vi "SequenceSelector_Load.vi"(0 "Ring 8":bool, 1 "Ring 7":bool, 2 "Ring 6":bool, 3 "Ring 5":bool, 4 "Loop Iteration":i32, 5 "Inflow Channel Selector":dbl, 7 "Ring 4":bool, 8 "Ring 3":bool, 9 "Ring 2":bool, 10 "Ring 1":bool) -> (6 "Array":u8[][](array[numeric])=[[0, 0, 0, 0, 0, 0, 0, 0, 2, 4, 3, 3, 3, 3], [0, 0, 0, 0, 0, 0, 0, 0, 0, 0, 0, 0, 0, 0], [0, 0, 0, 0, 0, 0, 0, 0, 0, 0, 0, 0, 0, 0], [0, 0, 0, 0, 0, 0, 0, 0, 0, 0, 0, 0, 0, 0], [0, 0, 0, 0, 0, 0, 0, 0, 0, 0, 0, 0, 0, 0], [11, 11, 11, 11, 11, 11, 11, 0, 0, 0, 0, 0, 0, 0], [0, 0, 0, 0, 0, 0, 0, 0, 0, 0, 0, 0, 0, 0], [16, 16, 16, 16, 16, 16, 16, 0, 0, 0, 0, 0, 0, 0], [0, 0, 0, 0, 0, 0, 0, 0, 0, 0, 0, 0, 0, 0], [0, 0, 0, 0, 0, 0, 0, 0, 0, 0, 0, 0, 0, 0], [0, 0, 0, 0, 0, 0, 0, 0, 0, 0, 0, 0, 0, 0], [2, 2, 2, 2, 2, 2, 2, 0, 0, 0, 0, 0, 0, 0], [4, 4, 4, 4, 4, 4, 4, 0, 0, 0, 0, 0, 0, 0], [255, 255, 255, 255, 255, 255, 0, 0, 0, 0, 0, 0, 0, 0], [3, 2, 6, 4, 5, 1, 0, 0, 0, 0, 0, 0, 0, 0], [31, 31, 31, 31, 31, 31, 0, 0, 0, 0, 0, 0, 0, 0], [255, 255, 255, 255, 255, 255, 0, 0, 0, 0, 0, 0, 0, 0]])   [LabVIEW 2016]
panel:
  in  "Byte 4":dbl[](array[numeric])
  in  "Byte 3":dbl[](array[numeric])
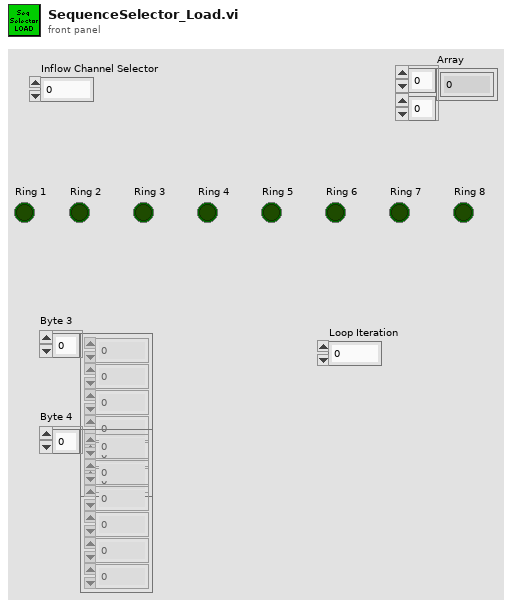
[diagram p1: front panel]
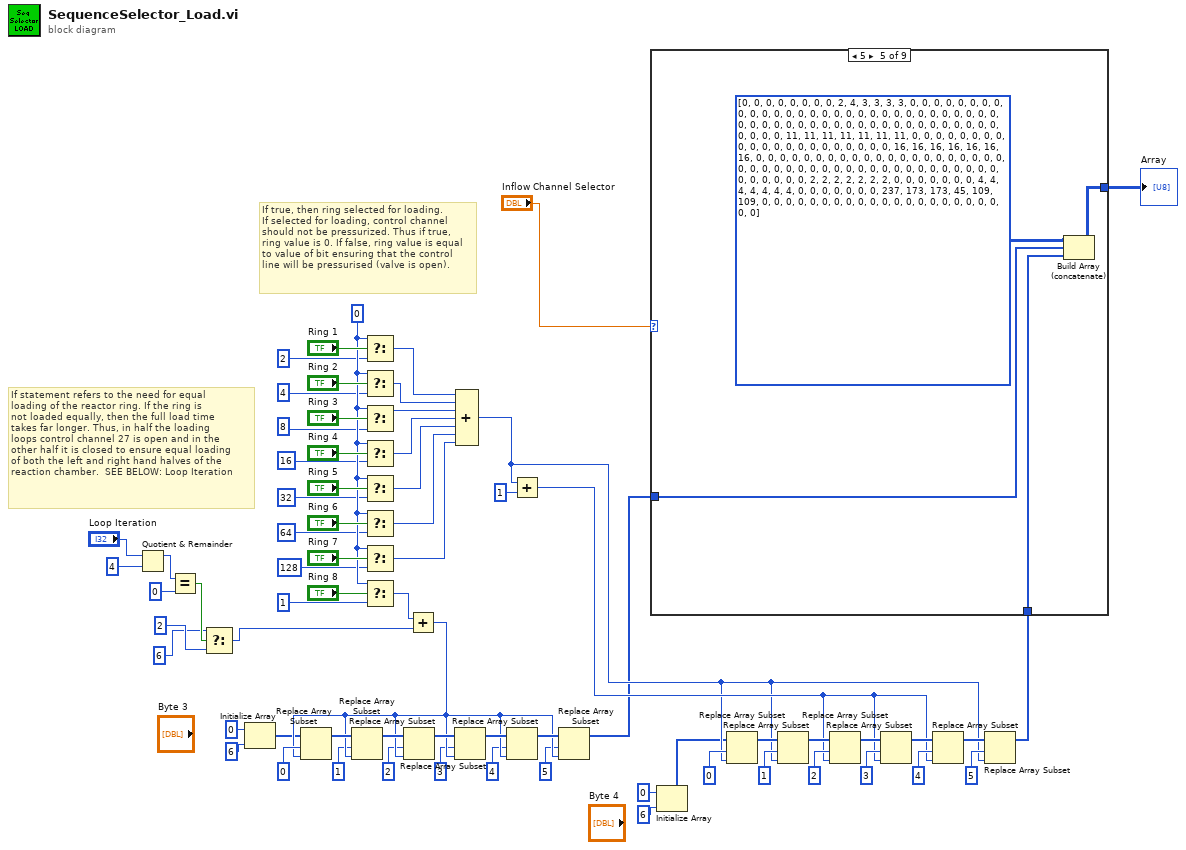
[diagram p0: block diagram]
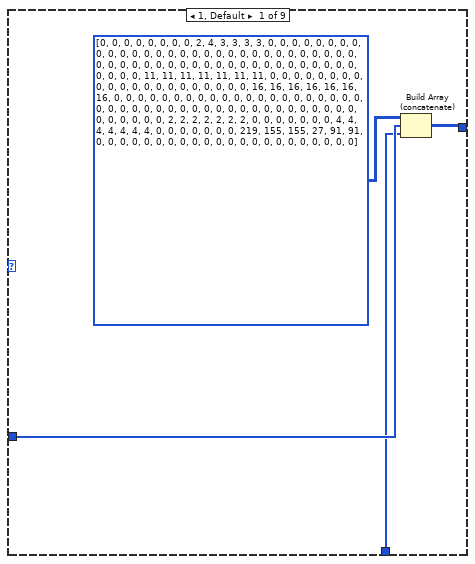
[diagram p2: hidden frame]
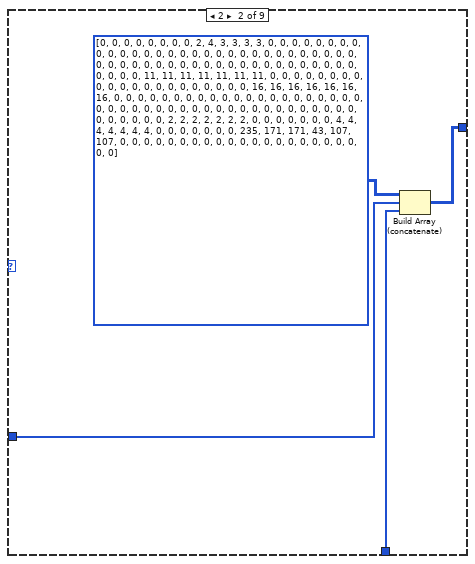
[diagram p3: hidden frame]
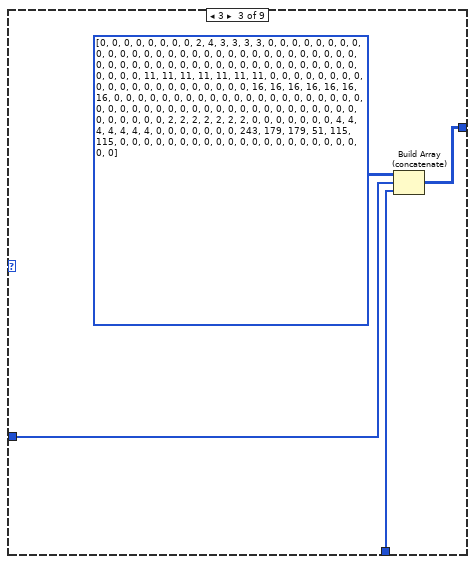
[diagram p4: hidden frame]
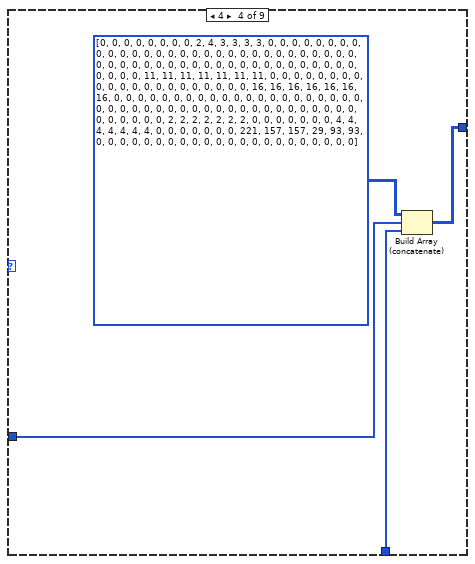
[diagram p5: hidden frame]
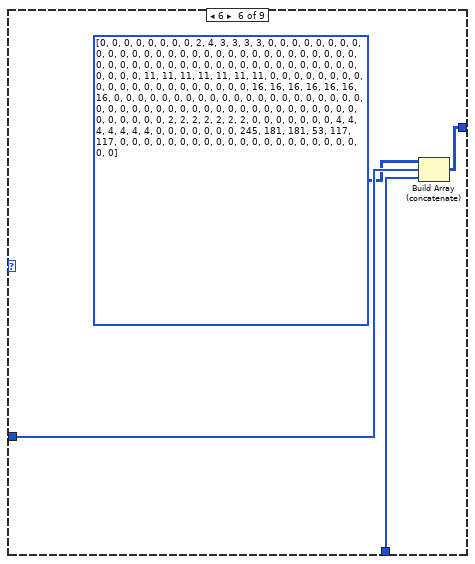
[diagram p6: hidden frame]
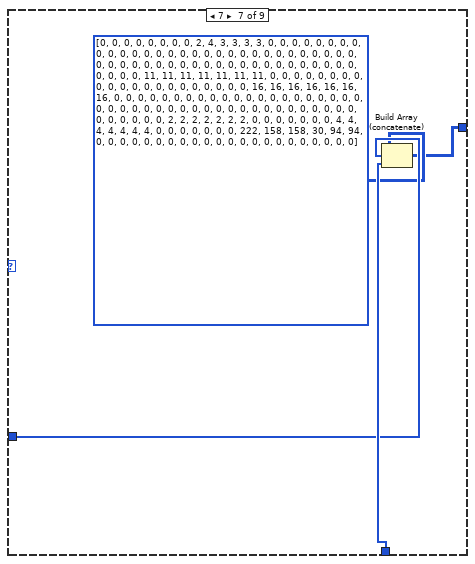
[diagram p7: hidden frame]
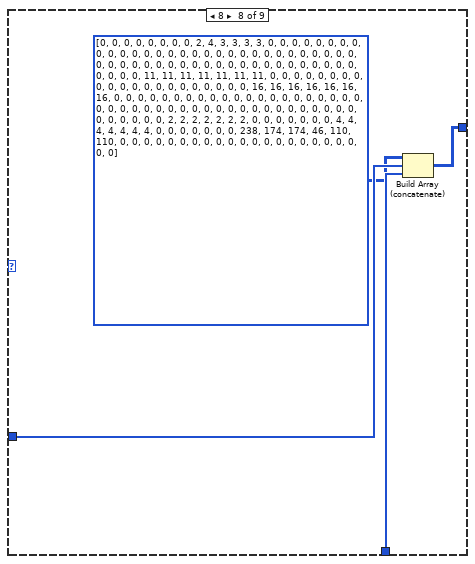
[diagram p8: hidden frame]
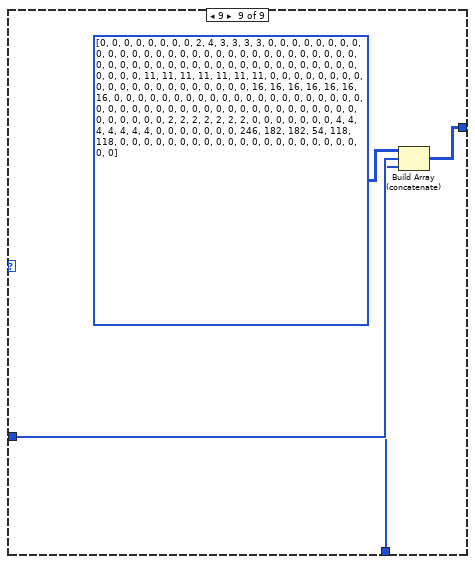
[diagram p9: hidden frame]
diagram:
  w60 = 0
  # "If statement refers to the need for equal \nloading of the reactor ring. If the ring is \nnot loaded equally, then the full load time \ntakes far longer. Thus, in half the loading\nloops control channel 27 is open and in the\nother half it is closed to ensure equal loading\nof both the left and right hand halves of the \nreaction chamber.  SEE BELOW: Loop Iteration"
  # "If true, then ring selected for loading. \nIf selected for loading, control channel\nshould not be pressurized. Thus if true, \nring value is 0. If false, ring value is equal\nto value of bit ensuring that the control \nline will be pressurised (valve is open)."
  n1 = Quotient & Remainder(x="Loop Iteration", y=4) -> (x-y*floor(x/y)=w4:i32)  [unwired: 1 out]
  n2 = Equal?(x=w4, y=0) -> (x = y?=w7:bool)
  n3 = Select(t=6, s=w7, f=2) -> (s? t:f=w8:i32)
  n4 = Initialize Array(0, 6) -> (w9:i32[])
  n5 = Select(t=w60, s="Ring 1", f=2) -> (s? t:f=w27:i32)
  n6 = Select(t=w60, s="Ring 2", f=4) -> (s? t:f=w26:i32)
  n7 = Select(t=w60, s="Ring 3", f=8) -> (s? t:f=w25:i32)
  n8 = Select(t=w60, s="Ring 4", f=16) -> (s? t:f=w24:i32)
  n9 = Select(t=w60, s="Ring 5", f=32) -> (s? t:f=w23:i32)
  n10 = Select(t=w60, s="Ring 6", f=64) -> (s? t:f=w22:i32)
  n11 = Select(t=w60, s="Ring 7", f=128) -> (s? t:f=w21:i32)
  n12 = Select(t=w60, s="Ring 8", f=1) -> (s? t:f=w51:i32)
  n13 = Add(x=w51, y=w8) -> (x+y=w44:i32)
  n14 = Replace Array Subset(array=w9, new element=w44, index=0) -> (w49:i32[])
  n15 = Replace Array Subset(array=w49, new element=w44, index=1) -> (w48:i32[])
  n16 = Replace Array Subset(array=w48, new element=w44, index=2) -> (w47:i32[])
  n17 = Replace Array Subset(array=w47, new element=w44, index=3) -> (w46:i32[])
  n18 = Compound Arithmetic op=ADD(w27, w26, w25, w24, w23, w22, w21) -> (w18:i32)
  n19 = Replace Array Subset(array=w46, new element=w44, index=4) -> (w45:i32[])
  n20 = Add(x=w18, y=1) -> (x+y=w19:i32)
  n21 = Replace Array Subset(array=w45, new element=w44, index=5) -> (w17:i32[])
  n22 = Initialize Array(0, 6) -> (w14:i32[])
  n23 = Replace Array Subset(array=w14, new element=w18, index=0) -> (w29:i32[])
  n24 = Replace Array Subset(array=w29, new element=w18, index=1) -> (w30:i32[])
  n25 = Replace Array Subset(array=w30, new element=w19, index=2) -> (w31:i32[])
  n26 = Replace Array Subset(array=w31, new element=w19, index=3) -> (w32:i32[])
  n27 = Replace Array Subset(array=w32, new element=w19, index=4) -> (w33:i32[])
  n28 = Replace Array Subset(array=w33, new element=w18, index=5) -> (w16:i32[])
  n29 = case shown="5" "Inflow Channel Selector" {
    tunnel: [w73 w74 w78 w82 w89 w93 w94 w98 w104] -> w15
    tunnel: w17 -> [w71 w76 w80 w84 w87 w91 w96 w100 w103]
    tunnel: w16 -> [w70 w77 w81 w85 w88 w92 w97 w101 w102]
    frame 1, Default {
      n30 = Build Array (concatenate)(u8[][] [[0, 0, 0, 0, 0, 0, 0, 0, 2, 4, 3, 3, 3, 3], [0, 0, 0, 0, 0, 0, 0, 0, 0, 0, 0, 0, 0, 0], [0, 0, 0, 0, 0, 0, 0, 0, 0, 0, 0, 0, 0, 0], [0, 0, 0, 0, 0, 0, 0, 0, 0, 0, 0, 0, 0, 0], [0, 0, 0, 0, 0, 0, 0, 0, 0, 0, 0, 0, 0, 0], [11, 11, 11, 11, 11, 11, 11, 0, 0, 0, 0, 0, 0, 0], [0, 0, 0, 0, 0, 0, 0, 0, 0, 0, 0, 0, 0, 0], [16, 16, 16, 16, 16, 16, 16, 0, 0, 0, 0, 0, 0, 0], [0, 0, 0, 0, 0, 0, 0, 0, 0, 0, 0, 0, 0, 0], [0, 0, 0, 0, 0, 0, 0, 0, 0, 0, 0, 0, 0, 0], [0, 0, 0, 0, 0, 0, 0, 0, 0, 0, 0, 0, 0, 0], [2, 2, 2, 2, 2, 2, 2, 0, 0, 0, 0, 0, 0, 0], [4, 4, 4, 4, 4, 4, 4, 0, 0, 0, 0, 0, 0, 0], [219, 155, 155, 27, 91, 91, 0, 0, 0, 0, 0, 0, 0, 0], [0, 0, 0, 0, 0, 0, 0, 0, 0, 0, 0, 0, 0, 0]], w71, w70) -> (w73:i32[][])
    }
    frame 2 {
      n31 = Build Array (concatenate)(u8[][] [[0, 0, 0, 0, 0, 0, 0, 0, 2, 4, 3, 3, 3, 3], [0, 0, 0, 0, 0, 0, 0, 0, 0, 0, 0, 0, 0, 0], [0, 0, 0, 0, 0, 0, 0, 0, 0, 0, 0, 0, 0, 0], [0, 0, 0, 0, 0, 0, 0, 0, 0, 0, 0, 0, 0, 0], [0, 0, 0, 0, 0, 0, 0, 0, 0, 0, 0, 0, 0, 0], [11, 11, 11, 11, 11, 11, 11, 0, 0, 0, 0, 0, 0, 0], [0, 0, 0, 0, 0, 0, 0, 0, 0, 0, 0, 0, 0, 0], [16, 16, 16, 16, 16, 16, 16, 0, 0, 0, 0, 0, 0, 0], [0, 0, 0, 0, 0, 0, 0, 0, 0, 0, 0, 0, 0, 0], [0, 0, 0, 0, 0, 0, 0, 0, 0, 0, 0, 0, 0, 0], [0, 0, 0, 0, 0, 0, 0, 0, 0, 0, 0, 0, 0, 0], [2, 2, 2, 2, 2, 2, 2, 0, 0, 0, 0, 0, 0, 0], [4, 4, 4, 4, 4, 4, 4, 0, 0, 0, 0, 0, 0, 0], [235, 171, 171, 43, 107, 107, 0, 0, 0, 0, 0, 0, 0, 0], [0, 0, 0, 0, 0, 0, 0, 0, 0, 0, 0, 0, 0, 0]], w76, w77) -> (w74:i32[][])
    }
    frame 3 {
      n32 = Build Array (concatenate)(u8[][] [[0, 0, 0, 0, 0, 0, 0, 0, 2, 4, 3, 3, 3, 3], [0, 0, 0, 0, 0, 0, 0, 0, 0, 0, 0, 0, 0, 0], [0, 0, 0, 0, 0, 0, 0, 0, 0, 0, 0, 0, 0, 0], [0, 0, 0, 0, 0, 0, 0, 0, 0, 0, 0, 0, 0, 0], [0, 0, 0, 0, 0, 0, 0, 0, 0, 0, 0, 0, 0, 0], [11, 11, 11, 11, 11, 11, 11, 0, 0, 0, 0, 0, 0, 0], [0, 0, 0, 0, 0, 0, 0, 0, 0, 0, 0, 0, 0, 0], [16, 16, 16, 16, 16, 16, 16, 0, 0, 0, 0, 0, 0, 0], [0, 0, 0, 0, 0, 0, 0, 0, 0, 0, 0, 0, 0, 0], [0, 0, 0, 0, 0, 0, 0, 0, 0, 0, 0, 0, 0, 0], [0, 0, 0, 0, 0, 0, 0, 0, 0, 0, 0, 0, 0, 0], [2, 2, 2, 2, 2, 2, 2, 0, 0, 0, 0, 0, 0, 0], [4, 4, 4, 4, 4, 4, 4, 0, 0, 0, 0, 0, 0, 0], [243, 179, 179, 51, 115, 115, 0, 0, 0, 0, 0, 0, 0, 0], [0, 0, 0, 0, 0, 0, 0, 0, 0, 0, 0, 0, 0, 0]], w80, w81) -> (w78:i32[][])
    }
    frame 4 {
      n33 = Build Array (concatenate)(u8[][] [[0, 0, 0, 0, 0, 0, 0, 0, 2, 4, 3, 3, 3, 3], [0, 0, 0, 0, 0, 0, 0, 0, 0, 0, 0, 0, 0, 0], [0, 0, 0, 0, 0, 0, 0, 0, 0, 0, 0, 0, 0, 0], [0, 0, 0, 0, 0, 0, 0, 0, 0, 0, 0, 0, 0, 0], [0, 0, 0, 0, 0, 0, 0, 0, 0, 0, 0, 0, 0, 0], [11, 11, 11, 11, 11, 11, 11, 0, 0, 0, 0, 0, 0, 0], [0, 0, 0, 0, 0, 0, 0, 0, 0, 0, 0, 0, 0, 0], [16, 16, 16, 16, 16, 16, 16, 0, 0, 0, 0, 0, 0, 0], [0, 0, 0, 0, 0, 0, 0, 0, 0, 0, 0, 0, 0, 0], [0, 0, 0, 0, 0, 0, 0, 0, 0, 0, 0, 0, 0, 0], [0, 0, 0, 0, 0, 0, 0, 0, 0, 0, 0, 0, 0, 0], [2, 2, 2, 2, 2, 2, 2, 0, 0, 0, 0, 0, 0, 0], [4, 4, 4, 4, 4, 4, 4, 0, 0, 0, 0, 0, 0, 0], [221, 157, 157, 29, 93, 93, 0, 0, 0, 0, 0, 0, 0, 0], [0, 0, 0, 0, 0, 0, 0, 0, 0, 0, 0, 0, 0, 0]], w84, w85) -> (w82:i32[][])
    }
    frame 5 {
      n34 = Build Array (concatenate)(u8[][] [[0, 0, 0, 0, 0, 0, 0, 0, 2, 4, 3, 3, 3, 3], [0, 0, 0, 0, 0, 0, 0, 0, 0, 0, 0, 0, 0, 0], [0, 0, 0, 0, 0, 0, 0, 0, 0, 0, 0, 0, 0, 0], [0, 0, 0, 0, 0, 0, 0, 0, 0, 0, 0, 0, 0, 0], [0, 0, 0, 0, 0, 0, 0, 0, 0, 0, 0, 0, 0, 0], [11, 11, 11, 11, 11, 11, 11, 0, 0, 0, 0, 0, 0, 0], [0, 0, 0, 0, 0, 0, 0, 0, 0, 0, 0, 0, 0, 0], [16, 16, 16, 16, 16, 16, 16, 0, 0, 0, 0, 0, 0, 0], [0, 0, 0, 0, 0, 0, 0, 0, 0, 0, 0, 0, 0, 0], [0, 0, 0, 0, 0, 0, 0, 0, 0, 0, 0, 0, 0, 0], [0, 0, 0, 0, 0, 0, 0, 0, 0, 0, 0, 0, 0, 0], [2, 2, 2, 2, 2, 2, 2, 0, 0, 0, 0, 0, 0, 0], [4, 4, 4, 4, 4, 4, 4, 0, 0, 0, 0, 0, 0, 0], [237, 173, 173, 45, 109, 109, 0, 0, 0, 0, 0, 0, 0, 0], [0, 0, 0, 0, 0, 0, 0, 0, 0, 0, 0, 0, 0, 0]], w87, w88) -> (w89:i32[][])
    }
    frame 6 {
      n35 = Build Array (concatenate)(u8[][] [[0, 0, 0, 0, 0, 0, 0, 0, 2, 4, 3, 3, 3, 3], [0, 0, 0, 0, 0, 0, 0, 0, 0, 0, 0, 0, 0, 0], [0, 0, 0, 0, 0, 0, 0, 0, 0, 0, 0, 0, 0, 0], [0, 0, 0, 0, 0, 0, 0, 0, 0, 0, 0, 0, 0, 0], [0, 0, 0, 0, 0, 0, 0, 0, 0, 0, 0, 0, 0, 0], [11, 11, 11, 11, 11, 11, 11, 0, 0, 0, 0, 0, 0, 0], [0, 0, 0, 0, 0, 0, 0, 0, 0, 0, 0, 0, 0, 0], [16, 16, 16, 16, 16, 16, 16, 0, 0, 0, 0, 0, 0, 0], [0, 0, 0, 0, 0, 0, 0, 0, 0, 0, 0, 0, 0, 0], [0, 0, 0, 0, 0, 0, 0, 0, 0, 0, 0, 0, 0, 0], [0, 0, 0, 0, 0, 0, 0, 0, 0, 0, 0, 0, 0, 0], [2, 2, 2, 2, 2, 2, 2, 0, 0, 0, 0, 0, 0, 0], [4, 4, 4, 4, 4, 4, 4, 0, 0, 0, 0, 0, 0, 0], [245, 181, 181, 53, 117, 117, 0, 0, 0, 0, 0, 0, 0, 0], [0, 0, 0, 0, 0, 0, 0, 0, 0, 0, 0, 0, 0, 0]], w91, w92) -> (w93:i32[][])
    }
    frame 7 {
      n36 = Build Array (concatenate)(u8[][] [[0, 0, 0, 0, 0, 0, 0, 0, 2, 4, 3, 3, 3, 3], [0, 0, 0, 0, 0, 0, 0, 0, 0, 0, 0, 0, 0, 0], [0, 0, 0, 0, 0, 0, 0, 0, 0, 0, 0, 0, 0, 0], [0, 0, 0, 0, 0, 0, 0, 0, 0, 0, 0, 0, 0, 0], [0, 0, 0, 0, 0, 0, 0, 0, 0, 0, 0, 0, 0, 0], [11, 11, 11, 11, 11, 11, 11, 0, 0, 0, 0, 0, 0, 0], [0, 0, 0, 0, 0, 0, 0, 0, 0, 0, 0, 0, 0, 0], [16, 16, 16, 16, 16, 16, 16, 0, 0, 0, 0, 0, 0, 0], [0, 0, 0, 0, 0, 0, 0, 0, 0, 0, 0, 0, 0, 0], [0, 0, 0, 0, 0, 0, 0, 0, 0, 0, 0, 0, 0, 0], [0, 0, 0, 0, 0, 0, 0, 0, 0, 0, 0, 0, 0, 0], [2, 2, 2, 2, 2, 2, 2, 0, 0, 0, 0, 0, 0, 0], [4, 4, 4, 4, 4, 4, 4, 0, 0, 0, 0, 0, 0, 0], [222, 158, 158, 30, 94, 94, 0, 0, 0, 0, 0, 0, 0, 0], [0, 0, 0, 0, 0, 0, 0, 0, 0, 0, 0, 0, 0, 0]], w96, w97) -> (w94:i32[][])
    }
    frame 8 {
      n37 = Build Array (concatenate)(u8[][] [[0, 0, 0, 0, 0, 0, 0, 0, 2, 4, 3, 3, 3, 3], [0, 0, 0, 0, 0, 0, 0, 0, 0, 0, 0, 0, 0, 0], [0, 0, 0, 0, 0, 0, 0, 0, 0, 0, 0, 0, 0, 0], [0, 0, 0, 0, 0, 0, 0, 0, 0, 0, 0, 0, 0, 0], [0, 0, 0, 0, 0, 0, 0, 0, 0, 0, 0, 0, 0, 0], [11, 11, 11, 11, 11, 11, 11, 0, 0, 0, 0, 0, 0, 0], [0, 0, 0, 0, 0, 0, 0, 0, 0, 0, 0, 0, 0, 0], [16, 16, 16, 16, 16, 16, 16, 0, 0, 0, 0, 0, 0, 0], [0, 0, 0, 0, 0, 0, 0, 0, 0, 0, 0, 0, 0, 0], [0, 0, 0, 0, 0, 0, 0, 0, 0, 0, 0, 0, 0, 0], [0, 0, 0, 0, 0, 0, 0, 0, 0, 0, 0, 0, 0, 0], [2, 2, 2, 2, 2, 2, 2, 0, 0, 0, 0, 0, 0, 0], [4, 4, 4, 4, 4, 4, 4, 0, 0, 0, 0, 0, 0, 0], [238, 174, 174, 46, 110, 110, 0, 0, 0, 0, 0, 0, 0, 0], [0, 0, 0, 0, 0, 0, 0, 0, 0, 0, 0, 0, 0, 0]], w100, w101) -> (w98:i32[][])
    }
    frame 9 {
      n38 = Build Array (concatenate)(u8[][] [[0, 0, 0, 0, 0, 0, 0, 0, 2, 4, 3, 3, 3, 3], [0, 0, 0, 0, 0, 0, 0, 0, 0, 0, 0, 0, 0, 0], [0, 0, 0, 0, 0, 0, 0, 0, 0, 0, 0, 0, 0, 0], [0, 0, 0, 0, 0, 0, 0, 0, 0, 0, 0, 0, 0, 0], [0, 0, 0, 0, 0, 0, 0, 0, 0, 0, 0, 0, 0, 0], [11, 11, 11, 11, 11, 11, 11, 0, 0, 0, 0, 0, 0, 0], [0, 0, 0, 0, 0, 0, 0, 0, 0, 0, 0, 0, 0, 0], [16, 16, 16, 16, 16, 16, 16, 0, 0, 0, 0, 0, 0, 0], [0, 0, 0, 0, 0, 0, 0, 0, 0, 0, 0, 0, 0, 0], [0, 0, 0, 0, 0, 0, 0, 0, 0, 0, 0, 0, 0, 0], [0, 0, 0, 0, 0, 0, 0, 0, 0, 0, 0, 0, 0, 0], [2, 2, 2, 2, 2, 2, 2, 0, 0, 0, 0, 0, 0, 0], [4, 4, 4, 4, 4, 4, 4, 0, 0, 0, 0, 0, 0, 0], [246, 182, 182, 54, 118, 118, 0, 0, 0, 0, 0, 0, 0, 0], [0, 0, 0, 0, 0, 0, 0, 0, 0, 0, 0, 0, 0, 0]], w103, w102) -> (w104:i32[][])
    }
  }
  "Array" <- w15
